vi "TIFF-Compute IFD Size.vi"(8 "[IN] Bits per sample":u32, 9 "[IN] Image width":u32, 10 "[IN] Image length":u32, 11 "[IN] Tags in IFD":u32=12) -> (1 "max frames":u32, 2 "[OUT] Image size in bytes":u32, 3 "[OUT] IFD size in bytes":u32)   [LabVIEW 2020]
doc: "This VI calculates the size of an image file directory (IFD)"
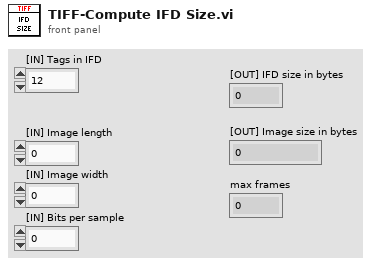
[diagram p1: front panel]
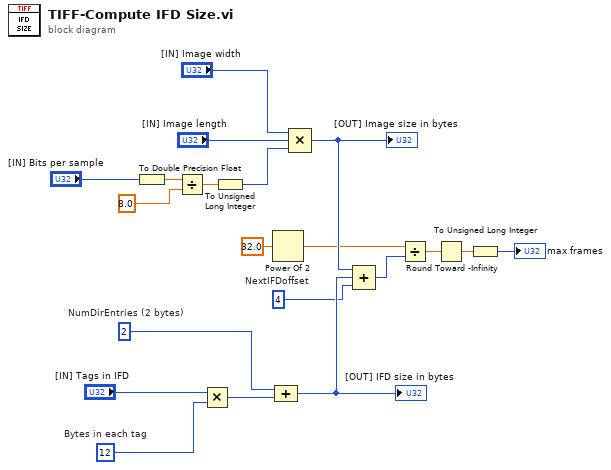
[diagram p0: block diagram]
diagram:
  w7 = u32 4  # NextIFDoffset
  w12 = u32 2  # NumDirEntries (2 bytes)
  w19 = u32 12  # Bytes in each tag
  n1 = To Double Precision Float(number="[IN] Bits per sample") -> (double precision float=w10:dbl)
  n2 = Divide(x=w10, y=8.0) -> (x/y=w17:dbl)
  n3 = Multiply(x="[IN] Tags in IFD", y=w19) -> (x*y=w18:u32)
  n4 = To Unsigned Long Integer(number=w17) -> (unsigned 32bit integer=w13:u32)
  n5 = Power Of 2(x=32.0) -> (2^x=w5:dbl)
  n6 = Compound Arithmetic op=ADD(w12, w18) -> (w8:u32)
  "[OUT] IFD size in bytes" <- w8
  n7 = Compound Arithmetic op=MULTIPLY("[IN] Image width", "[IN] Image length", w13) -> (w9:u32)
  "[OUT] Image size in bytes" <- w9
  n8 = Compound Arithmetic op=ADD(w9, w8, w7) -> (w4:u32)
  n9 = Divide(x=w5, y=w4) -> (x/y=w3:dbl)
  n10 = Round Toward -Infinity(1:w3) -> (0:w2:dbl)
  n11 = To Unsigned Long Integer(number=w2) -> (unsigned 32bit integer=→"max frames":u32)
